vi "StopALL.vi"(8 "error in (no error)":errorcluster, 11 "Queue References In":T1) -> (0 "error out":errorcluster, 3 "Queue ReferencesOut":T1)   [LabVIEW 2014, in "QueueMaintenance.lvlib"]
doc: "QSM Initialization:\n\nMultiple initialization steps are triggered by this VI before 'entering' the associated loops. Each initialization is intended for functions required be the first user event is available."
uses:
  QueueMaintenance.lvlib
  TypeDef/QSMRef_ALL.ctl
  Queue_TESTGUIUPDATE/Controls/QSM_Reference.ctl
  Queue_TESTGUIUPDATE/Controls/QSM_DataType.ctl
  Queue_TESTGUIUPDATE/Controls/QSM_RunStates.ctl
  Queue_TEST/Controls/QSM_Reference.ctl
  Queue_TEST/Controls/QSM_DataType.ctl
  Queue_TEST/Controls/QSM_RunStates.ctl
  Queue_TESTGUIUPDATE/GUIUpdateQSM.lvlib
  Queue_TEST/TestQSM.lvlib
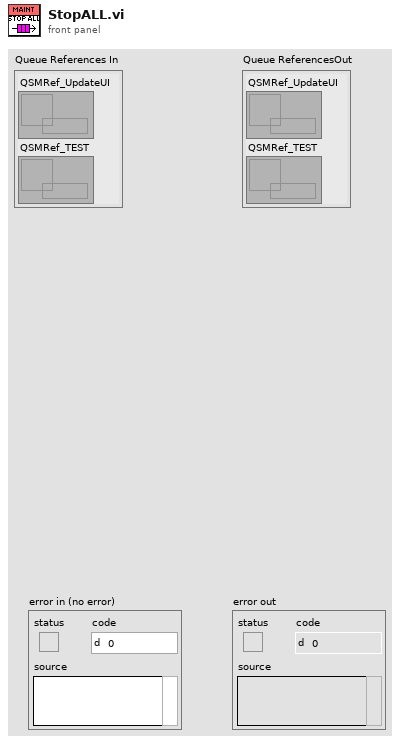
[diagram p1: front panel]
types:
  T1 = typedef "QueueMaintenance.lvlib/QSMRef_ALL.ctl" = cluster{"QSMRef_UpdateUI":T2, "QSMRef_TEST":T3}
  T2 = typedef "GUIUpdateQSM.lvlib/QSM_Reference.ctl" = refnum<queue>
  T3 = typedef "TestQSM.lvlib/QSM_Reference.ctl" = refnum<queue>
  T4 = typedef "TestQSM.lvlib/QSM_RunStates.ctl" = enum16{"NULL", "Sect01-Initialize-00-GROUP.ENQUEUE", "Sect02-Single File_Check for Parameters", "Sect02-Single File_Ask for File", "Sect02-Single File_Run Analysis", "Sect02-Single File_Write Results", "Sect03-Single ROI Calc_Check for Parameters", "Sect03-Single ROI Calc_Ask for File", "Sect03-Single ROI Calc_Run Analysis", "Sect03-Single ROI _Write Results", "Sect12-Full Dir_Check for Parameters", "Sect12-Full Dir_Ask for Dir", "Sect12-Full Dir_Check for Next Image to Process", "Sect12-Full Dir_Run Analysis", "Sect12-Full Dir_Write Results", "Sect12-Full Dir_Check if User Stopped", "Sect13-FullDir ROI Calc_Check for Parameters", "Sect13-FullDir ROI Calc_Ask for Dir", "Sect13-Full Dir ROI Calc_Check for Next Image to Process", "Sect13-Full Dir ROI Calc_Run Analysis", "Sect13-Full Dir ROI Calc_Write Results", "Sect13-Full Dir ROI Calc_Check if User Stopped", "Sect90-GUI_Config_Change UI Before Analysis", "Sect90-GUI_Config_Change UI After Analysis", "Sect90-GUI_Stop Processing Pressed", "Sect90-GUI_Stop Processing Button Set Back to F", "Sect90-GUI_Clear ROIs", "Sect99_EXIT-00-Group.Enqueue", "Sect99_EXIT-01-StopQSM"}
  T5 = typedef "GUIUpdateQSM.lvlib/QSM_RunStates.ctl" = enum16{"NULL", "Sect01_Initialize-00_GROUP.ENQUEUE", "Sect01_Initialize-01_SetMainToDefault", "Sect01_Initialize-02_Clear Status Strings", "Sect02_UpdateUI-00_Enable Stop_ Disable Start", "Sect02_UpdateUI-01_Enable Start_Disable Stop", "Sect02_UpdateUI-02_Update Status String", "Sect02_UpdateUI-03_Clear XY-Graph", "Sect03-Open ROI  GUI", "Sect03-Close ROI GUI", "Sect99_EXIT-00_Group.Enqueue", "Sect99_EXIT-01_CloseReferences", "Sect99_EXIT-02_StopQSM"}
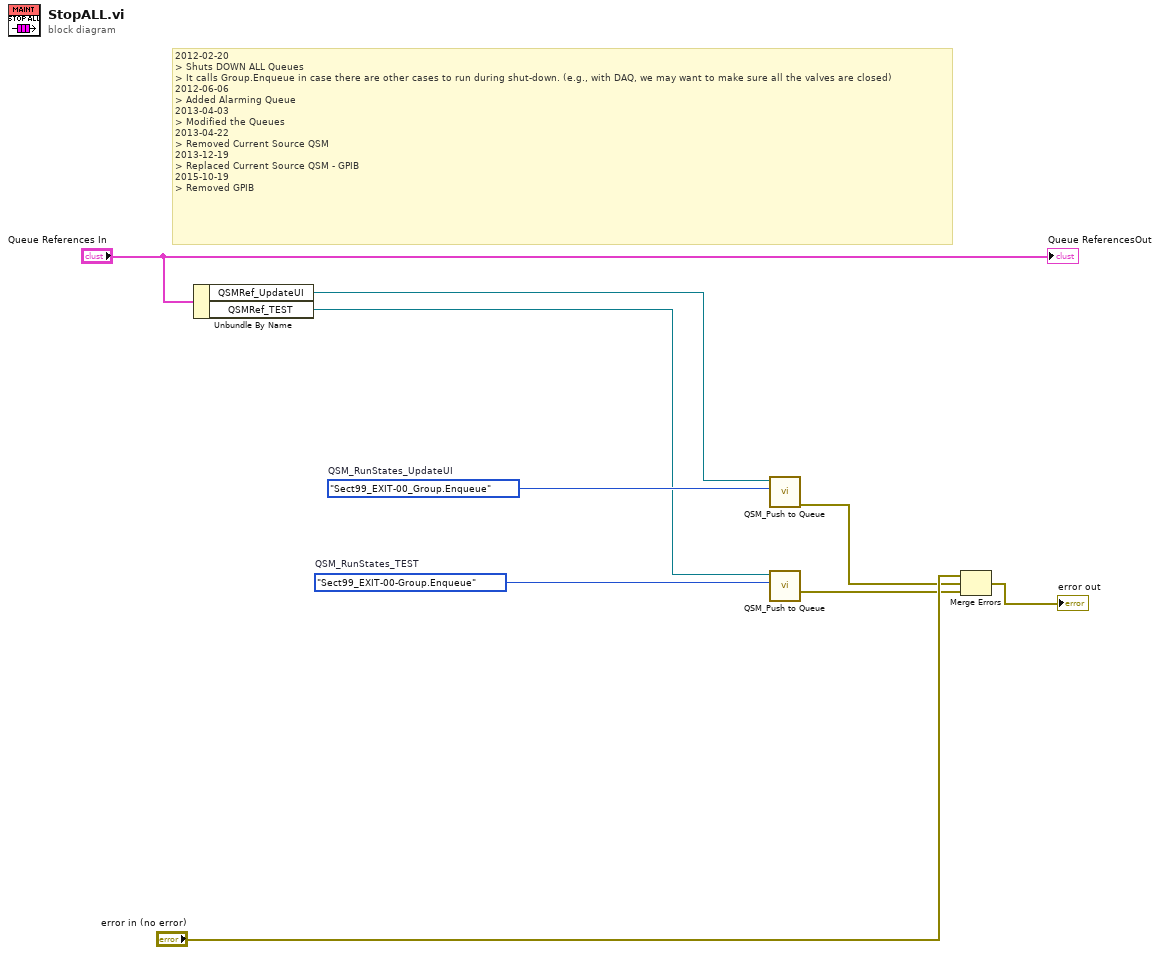
[diagram p0: block diagram]
diagram:
  w4 = QSM_RunStates."Sect99_EXIT-00-Group.Enqueue"  # QSM_RunStates_TEST
  w8 = QSM_RunStates."Sect99_EXIT-00_Group.Enqueue"  # QSM_RunStates_UpdateUI
  # "2012-02-20\n> Shuts DOWN ALL Queues\n> It calls Group.Enqueue in case there are other cases to run during shut-down. (e.g., with DAQ, we may want to make sure all the valves are closed)\n2012-06-06\n> Added Alarming Queue\n2013-04-03\n> Modified the Queues\n2013-04-22\n> Removed Current Source QSM\n2013-12-19\n> Replaced Current Source QSM - GPIB\n2015-10-19\n> Removed GPIB"
  n1 = Unbundle By Name("Queue References In") -> ("QSMRef_UpdateUI"=w9:T2, "QSMRef_TEST"=w5:T3)
  n2 = call "QSM_Push to Queue.vi"("QSM_RunStates"=w8, "QSMRef in"=w9) -> ("error out"=w2:errorcluster)  [unwired: 8 in, 1 out]
  n3 = call "QSM_Push to Queue.vi"("QSM_RunStates_TEST"=w4, "QSM_Reference_TEST"=w5) -> ("error out"=w1:errorcluster)  [unwired: 8 in, 1 out]
  n4 = Merge Errors("error in (no error)", w2, w1) -> (→"error out":errorcluster)
  "Queue ReferencesOut" <- "Queue References In"
